vi "SetAxisAcceleration.vi"(8 "error in (no error)":errorcluster, 10 "Acceleration":i32, 11 "Picomoto8742ControllerClass in":refnum<class "Picomoto8742ControllerClass.lvclass">) -> (0 "error out":errorcluster, 2 "Success?":bool, 3 "Picomoto8742ControllerClass out":refnum<class "Picomoto8742ControllerClass.lvclass">)   [LabVIEW 2020, in "Picomoto8742ControllerClass.lvclass"]
doc: "Send the acceleration setting relative to the active axis, to the physical device"
uses:
  Picomoto8742ControllerClass.lvclass
  Picomoto8742ControllerClass.lvclass/Picomoto8742ControllerClass.ctl
  PicoMotor8742Axis/Picomotor8742Axis.lvclass
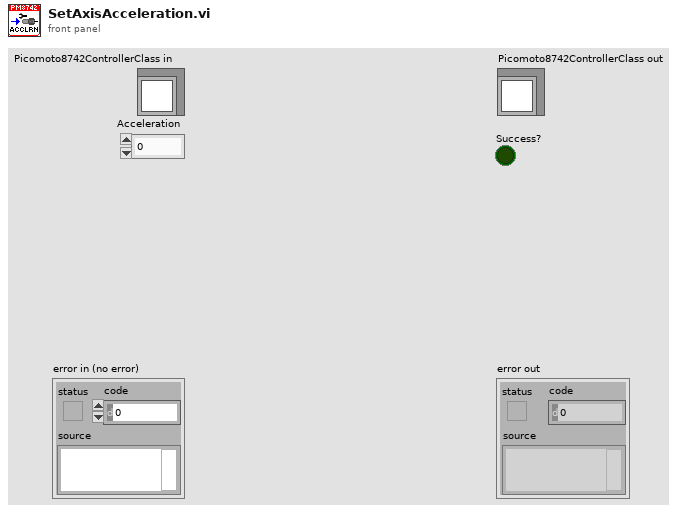
[diagram p1: front panel]
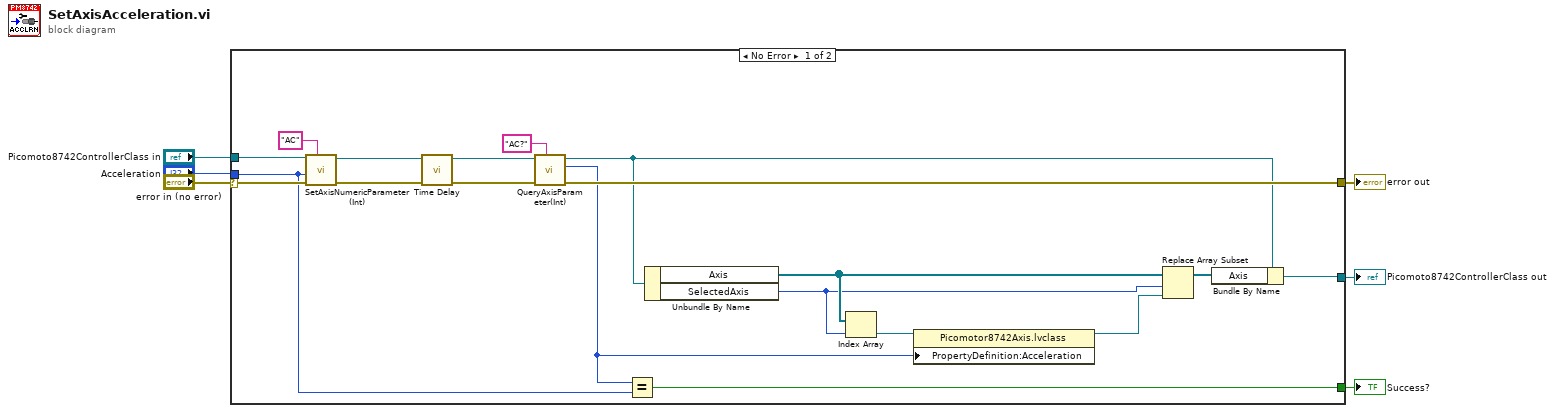
[diagram p0: block diagram]
diagram:
  n1 = case shown="No Error" "error in (no error)" {
    selector: "error in (no error)" -> [w24 w26]
    tunnel: [w23 w26] -> w5
    tunnel: [w20 w25] -> w3
    tunnel: "Picomoto8742ControllerClass in" -> [w19 w25]
    tunnel: "Acceleration" -> [w8 _]
    tunnel: [w7 _] -> w1
    frame No Error {
      n2 = call "SetAxisNumericParameter(Int).vi"("CMD"="AC" ("string"), "error in (no error)"=w24, "ParameterValue"=w8, "Picomoto8742ControllerClass in"=w19) -> ("error out"=w11:errorcluster, "Picomoto8742ControllerClass Out"=w16:refnum<class "Picomoto8742ControllerClass.lvclass">)  [unwired: 6 in]
      n3 = call "Time Delay"("error in (no error)"=w11) -> ("error out"=w10:errorcluster)  [unwired: 10 in]
      n4 = call-dynamic "QueryAxisParameter(Int).vi"("Cmd"="AC?" ("string"), "error in (no error)"=w10, "Picomoto8742ControllerClass in"=w16) -> ("error out"=w23:errorcluster, "ValueOut"=w9:i32, "Picomoto8742ControllerClass Out"=w12:refnum<class "Picomoto8742ControllerClass.lvclass">)  [unwired: 6 in]
      n5 = Equal?(x=w9, y=w8) -> (x = y?=w7:bool)
      n6 = Unbundle By Name(w12) -> ("Axis"=w15:refnum<class "Picomotor8742Axis.lvclass">[], "SelectedAxis"=w14:u32)
      n7 = Index Array(array=w15, index=w14) -> (element=w13:refnum<class "Picomotor8742Axis.lvclass">)
      n8 = property class="Picomotor8742Axis.lvclass"(reference=w13, "PropertyDefinition:Acceleration"=w9) -> (reference out=w22:refnum<class "Picomotor8742Axis.lvclass">)  [unwired: 1 in, 1 out]
      n9 = Replace Array Subset(array=w15, new element=w22, index=w14) -> (w21:refnum<class "Picomotor8742Axis.lvclass">[])
      n10 = Bundle By Name(cluster=w12, "Axis"=w21) -> (w20:refnum<class "Picomoto8742ControllerClass.lvclass">)
    }
    frame Error {
    }
  }
  "error out" <- w5
  "Picomoto8742ControllerClass out" <- w3
  "Success?" <- w1
